vi "comm get port name.vi"(8 "error in (no error)":errorcluster, 11 "Comm Handle":u64) -> (0 "error out":errorcluster, 1 "original port name":string, 2 "port name":string, 3 "dup Comm Handle":u64)   [LabVIEW 2009, in "lvserial.lvlib"]
doc: "Retrieves the name of the serial port."
uses:
  lvserial.lvlib
  x64/Release/lvserial.dll
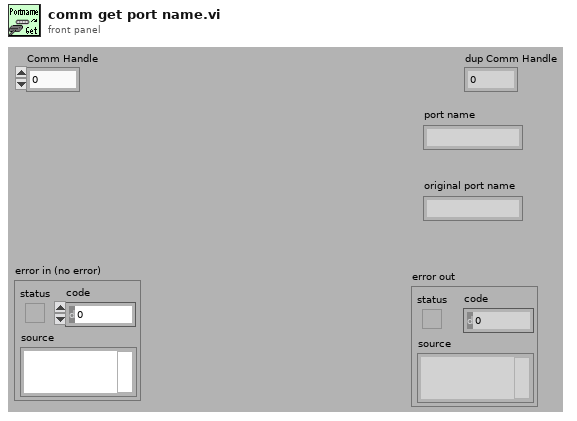
[diagram p1: front panel]
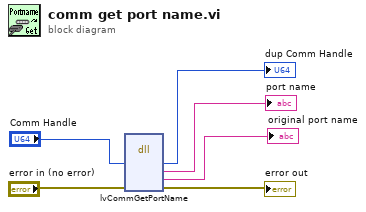
[diagram p0: block diagram]
diagram:
  n1 = dll-call lib="C:/Users/Admin/Desktop/lvserial_source_1-2-13/x64/Release/lvserial.dll" fn="lvCommGetPortName"("hComm"="Comm Handle", "pError"="error in (no error)") -> ("hComm"=→"dup Comm Handle":u64, "shName"=→"port name":string, "shOriginal"=→"original port name":string, "pError"=→"error out":errorcluster)  [unwired: 4 in, 4 out]
